vi "Brute Force Measurment SubVI.vi"(0 "Pins In":refnum<k21>[](array[refnum]), 4 "Barcodes in":string[](array[string]), 5 "Channel # in":i32, 6 "Last Tube #":i32, 7 "error in (no error)":errorcluster, 9 "BoardHandle in":T1) -> (11 "Actual Voltage Level (V) 2":dbl format="%#_13g", 12 "Individual Tube Current (Nano Amps)":dbl[](array[numeric]), 13 "Failed Tubes":string[](array[string]), 14 "Pins Out":refnum<k21>[](array[refnum]), 18 "error out":errorcluster, 19 "BoardHandle out":T1)   [LabVIEW 2020]
panel:
  # "Pin in."
  # "Output pin positions"
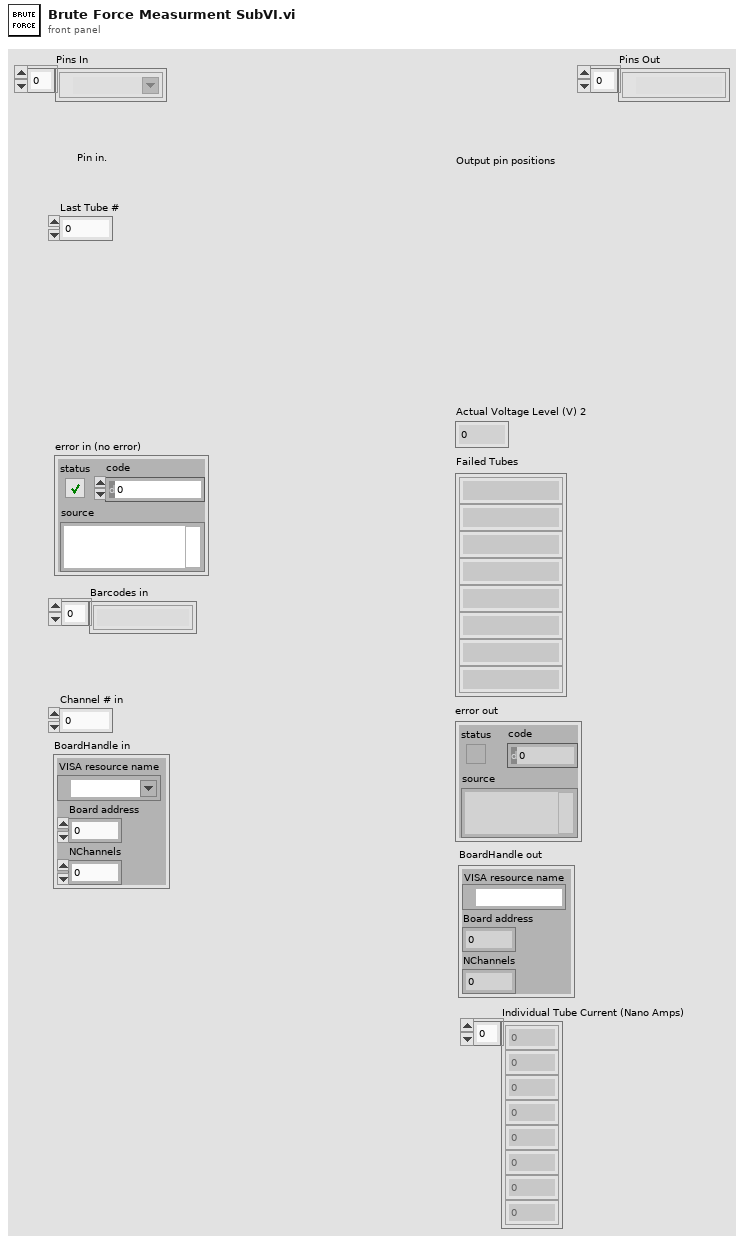
[diagram p1: front panel]
types:
  T1 = cluster{"VISA resource name":refnum<visa-resource-name>, "Board address":u8, "NChannels":u8}
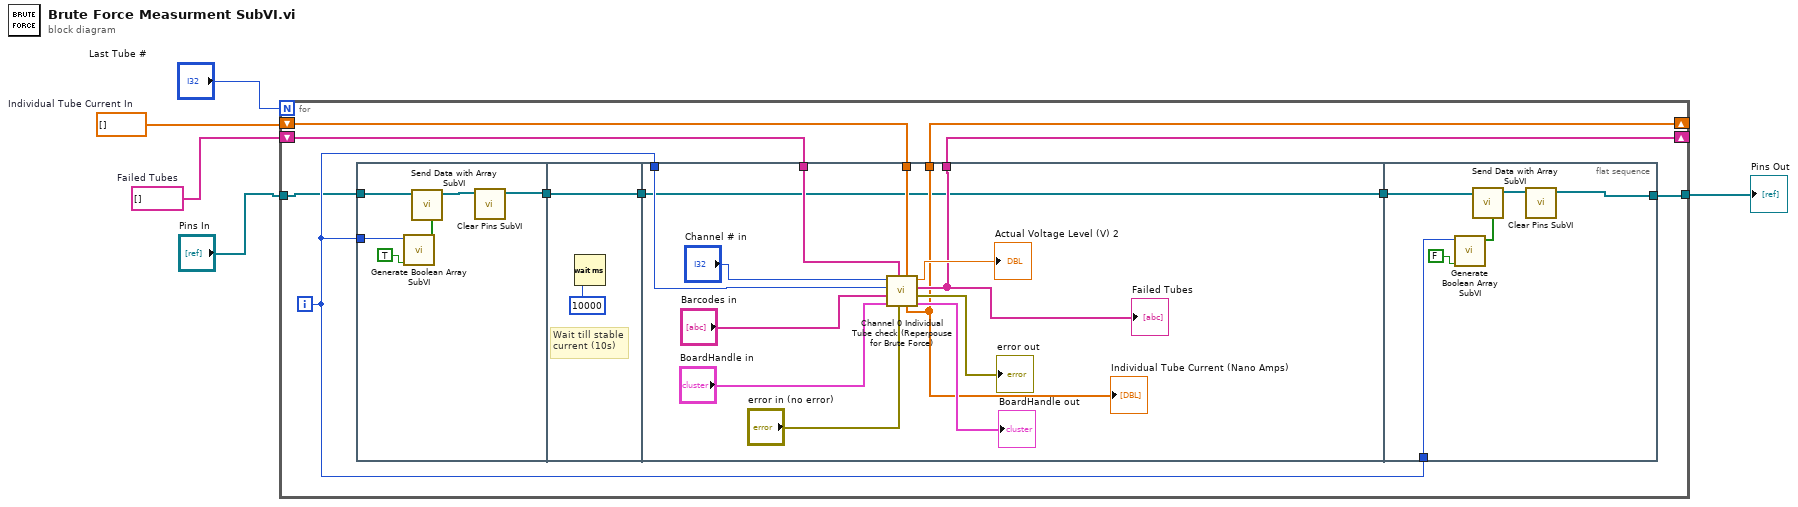
[diagram p0: block diagram]
diagram:
  w3 = dbl[] []  # Individual Tube Current In
  w4 = string[] []  # Failed Tubes
  n1 = for {
    N: "Last Tube #" -> [_]
    shift-right: [w13] -> _
    shift-left: w4 -> [w14]
    shift-right: [w11] -> _
    shift-left: w3 -> [w12]
    tunnel: "Pins In" -> [w10]
    tunnel: [w6] -> w1
    i -> [w15]
    n2 = flat-sequence {
      tunnel: [w20] -> w7
      tunnel: w10 -> [w16]
      tunnel: w15 -> [w19]
      tunnel: [w22] -> w8
      tunnel: w7 -> [w22]
      tunnel: w15 -> [w29]
      tunnel: w14 -> [w28]
      tunnel: [w27] -> w13
      tunnel: w12 -> [w26]
      tunnel: [w25] -> w11
      tunnel: [w24] -> w9
      tunnel: w8 -> [w24]
      tunnel: [w41] -> w6
      tunnel: w9 -> [w37]
      tunnel: w15 -> [w40]
      frame #0 {
        n3 = call "Generate Boolean Array SubVI.vi"("Activate: 1\nDeactivate: 0"=TRUE, "Tube"=w19) -> ("Boolean array"=w17:bool[])  [unwired: 9 in]
        n4 = call "Send Data with Array SubVI.vi"("Pins In"=w16, "Data"=w17) -> ("Pins Out"=w21:refnum<k21>[])  [unwired: 7 in]
        n5 = call "Clear Pins SubVI.vi"("Pins In"=w21) -> ("Pins Out"=w20:refnum<k21>[])  [unwired: 10 in]
      }
      frame #1 {
        # "Wait till stable\ncurrent (10s)"
        n6 = Wait (ms)(milliseconds to wait=u32 10000) -> ()  [unwired: 1 out]
      }
      frame #2 {
        n7 = call "Channel 0 Individual Tube check (Reperpouse for Brute Force).vi"("Individual Tube Current In"=w26, "error in (no error)"="error in (no error)", "Failed Tubes In"=w28, "BoardHandle in"="BoardHandle in", "Barcodes in"="Barcodes in", "Tube #"=w29, "Channel # in"="Channel # in") -> ("BoardHandle out"=→"BoardHandle out":T1, "error out"=→"error out":errorcluster, "Failed Tubes"=w27:string[], "Actual Voltage Level (V) 2"=→"Actual Voltage Level (V) 2":dbl, "Individual Tube Current (Nano Amps)"=w25:dbl[])
        "Failed Tubes" <- w27
        "Individual Tube Current (Nano Amps)" <- w25
      }
      frame #3 {
        n8 = call "Generate Boolean Array SubVI.vi"("Activate: 1\nDeactivate: 0"=FALSE, "Tube"=w40) -> ("Boolean array"=w38:bool[])  [unwired: 9 in]
        n9 = call "Send Data with Array SubVI.vi"("Pins In"=w37, "Data"=w38) -> ("Pins Out"=w42:refnum<k21>[])  [unwired: 7 in]
        n10 = call "Clear Pins SubVI.vi"("Pins In"=w42) -> ("Pins Out"=w41:refnum<k21>[])  [unwired: 10 in]
      }
    }
  }
  "Pins Out" <- w1
